vi "Self Test.vi"(8 "error in (no error)":errorcluster, 11 "Yokogawa AQ6370D in":refnum<class "Yokogawa AQ6370D.lvclass">) -> (0 "error out":errorcluster, 2 "Response":string, 3 "Yokogawa AQ6370D out":refnum<class "Yokogawa AQ6370D.lvclass">)   [LabVIEW 2018, in "Yokogawa AQ6370D.lvlib" / "Yokogawa AQ6370D.lvclass"]
uses:
  Yokogawa AQ6370D.lvclass
  Yokogawa AQ6370D.lvclass/Yokogawa AQ6370D.ctl
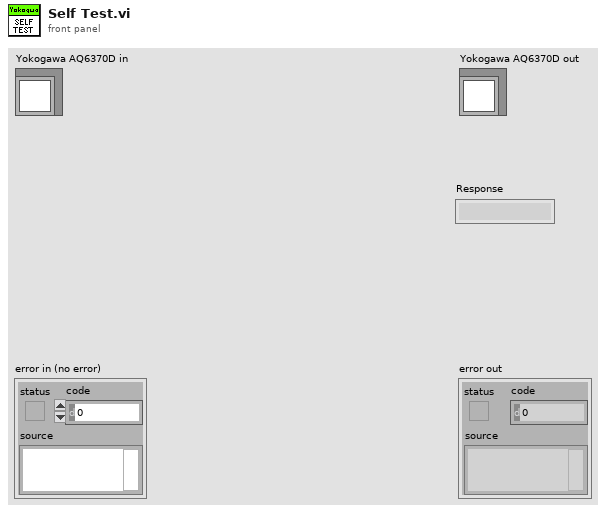
[diagram p1: front panel]
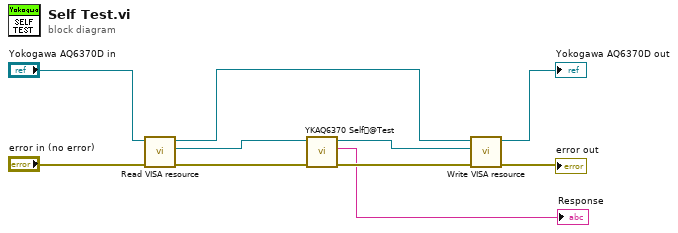
[diagram p0: block diagram]
diagram:
  n1 = call "Read VISA resource.vi"("error in (no error)"="error in (no error)", "Yokogawa AQ6370D in"="Yokogawa AQ6370D in") -> ("error out"=w9:errorcluster, "VISA resource"=w3:refnum<visa-resource-name>, "Yokogawa AQ6370D out"=w6:refnum<class "Yokogawa AQ6370D.lvclass">)  [unwired: 7 in]
  n2 = call "YKAQ6370 Self@Test.vi"("error in (no error)"=w9, "VISA resource name"=w3) -> ("error out"=w8:errorcluster, "Self-Test Response"=→"Response":string, "VISA resource name out"=w5:refnum<visa-resource-name>)  [unwired: 7 in]
  n3 = call "Write VISA resource.vi"("error in (no error)"=w8, "VISA resource"=w5, "Yokogawa AQ6370D in"=w6) -> ("error out"=→"error out":errorcluster, "Yokogawa AQ6370D out"=→"Yokogawa AQ6370D out":refnum<class "Yokogawa AQ6370D.lvclass">)  [unwired: 7 in]
